vi "DP41 Main.vi"() -> ()   [LabVIEW 2016]
panel:
  out "Data Stream 5":string
  out "Data Stream 4":string
  out "Data Stream 3":string
  out "(hi.lo)":u16
  in  "lo":u8 format="%x"
  in  "hi":u8 format="%x"
  in  "Numeric":u8 format="%.0x"
  out "unsigned byte array 2":u8[](array[numeric]) format="%.0x"
  in  "Data Stream 2":string
  out "unsigned byte array":u8[](array[numeric]) format="%.0x"
  in  "VISA Refnum in":refnum<visa-resource-name>
  out "Data Stream":string
  in  "Command Write":string
  in  "stop":bool
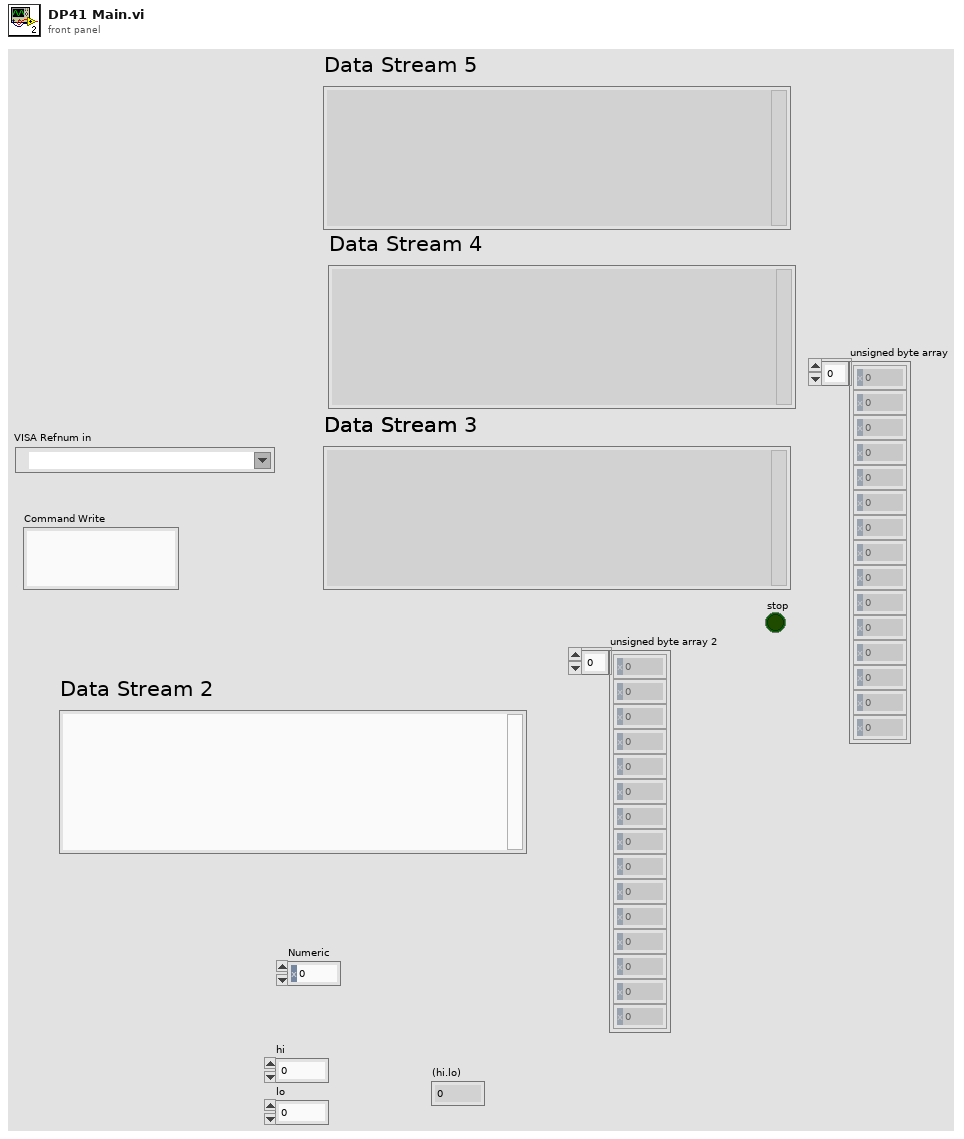
[diagram p1: front panel]
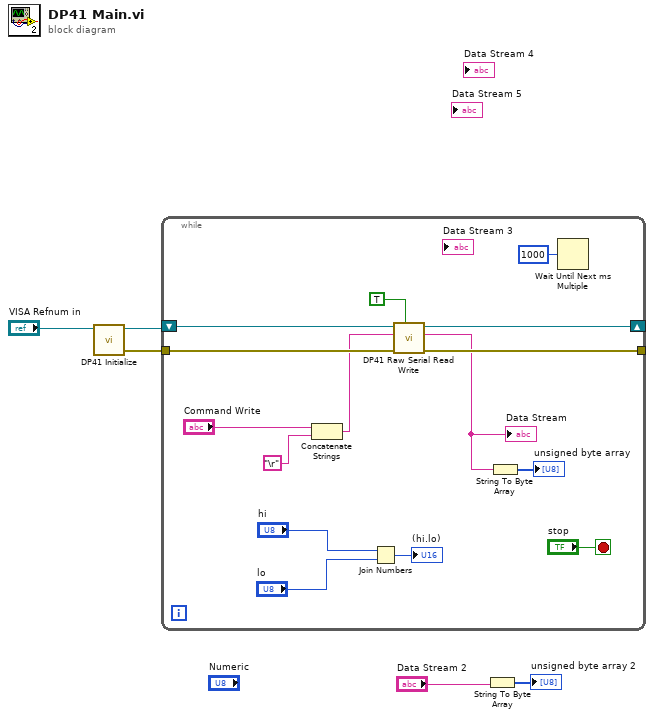
[diagram p0: block diagram]
diagram:
  n1 = call "DP41 Initialize.vi"("VISA Refnum in"="VISA Refnum in") -> ("error out"=w5:errorcluster, "VISA Refnum out"=w4:refnum<visa-resource-name>)  [unwired: 9 in]
  n2 = while {
    tunnel: w5 -> [w20]
    shift-right: [w18] -> _
    shift-left: w4 -> [w19]
    tunnel: [w17] -> _
    stop <- "stop" stop-if-true
    n3 = Concatenate Strings("Command Write", "\r") -> (w12:string)
    n4 = Join Numbers(hi="hi", lo="lo") -> ((hi.lo)=→"(hi.lo)":u16)
    n5 = call "DP41 Raw Serial Read Write.vi"("Read Only?"=TRUE, "error in (no error)"=w20, "Command Write"=w12, "VISA Refnum in"=w19) -> ("error out"=w17:errorcluster, "Data Stream"=w10:string, "VISA Refnum out"=w18:refnum<visa-resource-name>)  [unwired: 5 in]
    "Data Stream" <- w10
    n6 = String To Byte Array(string=w10) -> (unsigned byte array=→"unsigned byte array":u8[])
    n7 = Wait Until Next ms Multiple(millisecond multiple=u32 1000) -> ()  [unwired: 1 out]
  }
  n8 = String To Byte Array(string="Data Stream 2") -> (unsigned byte array=→"unsigned byte array 2":u8[])
